vi "数据存储表格-2.vi"(1 "循环次数":dbl, 2 "数组":dbl[](array[numeric]), 3 "频率":dbl, 4 "file path (dialog if empty)":path caption="文件路径 （空时为对话框）") -> (0 "采样时间":dbl)   [LabVIEW 2018]
uses:
  <vilib>/Utility/file.llb/Write Delimited Spreadsheet (DBL).vi
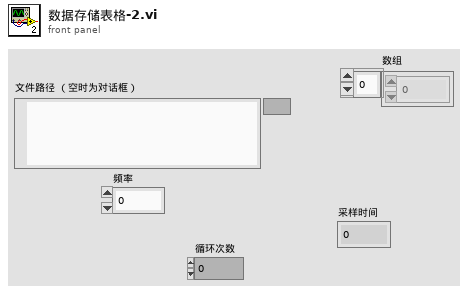
[diagram p1: front panel]
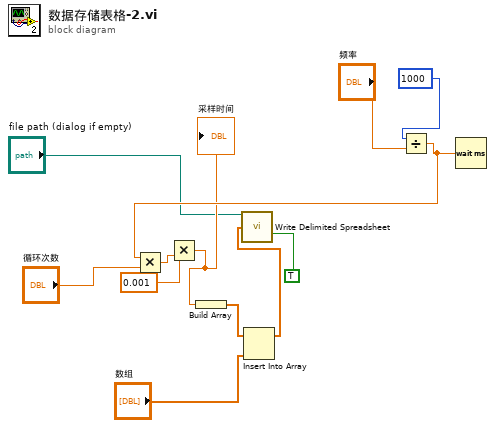
[diagram p0: block diagram]
diagram:
  n1 = Divide(x=1000, y="频率") -> (x/y=w9:dbl)
  n2 = Multiply(x=w9, y="循环次数") -> (x*y=w8:dbl)
  n3 = Multiply(x=0.001, y=w8) -> (x*y=w6:dbl)
  "采样时间" <- w6
  n4 = Build Array(w6) -> (w3:dbl[])
  n5 = Insert Into Array(array=w3, new element="数组") -> (w2:dbl[])  [unwired: 1 in]
  n6 = call-poly <vilib>:"Write Delimited Spreadsheet.vi"("file path (dialog if empty)"="file path (dialog if empty)", "1D data"=w2, "append to file? (new file:F)"=TRUE) -> ()  [unwired: 11 in, 2 out]
  n7 = Wait (ms)(milliseconds to wait=w9) -> ()  [unwired: 1 out]
